vi "Duplicate.vi"(8 "error in":errorcluster, 10 "parameters":variant, 11 "DMM Channel in":refnum<class "DMM Channel.lvclass">) -> (0 "error out":errorcluster, 3 "DMM Channel out":refnum<class "DMM Channel.lvclass">)   [LabVIEW 2025, in "DMM.lvlib" / "DMM Channel.lvclass"]
doc: "Implements the specific behavior of a node when it is being duplicated\nCan be used to change the name of the new node for example adding Copy to it. \nCopyright 2017 National Instruments Corporation\n\nLicensed under the Apache License, Version 2.0 (the \"License\"); you may not use this file except in compliance with the License. You may obtain a copy of the License at http://www.apache.org/licenses/LICENSE-2.0\nUnless required by applicable law or agreed to in writing, software distributed under the License is distributed on an \"AS IS\" BASIS, WITHOUT WARRANTIES OR CONDITIONS OF ANY KIND, either express or implied. See the License for the specific language governing permissions and limitations under the License."
uses:
  DMM Channel.lvclass
  DMM Channel.lvclass/DMM Channel.ctl
  Users/Public/Documents/Sandia National Labs/TSS Plugin/Abstract Engine.lvlibp/Plugin/Abstract/Channel configuration/Read Channel Setting.vi
  Users/Public/Documents/Sandia National Labs/TSS Plugin/Abstract Engine.lvlibp/Plugin/Abstract/Channel configuration/Write Channel Setting.vi
  Users/Public/Documents/Sandia National Labs/TSS Plugin/Abstract Engine.lvlibp/Plugin/Abstract/Abstract Channel/Abstract Channel.lvclass
  Users/Public/Documents/Sandia National Labs/TSS Plugin/Abstract Engine.lvlibp/Plugin/Abstract/Channel configuration/Channel configuration.lvclass
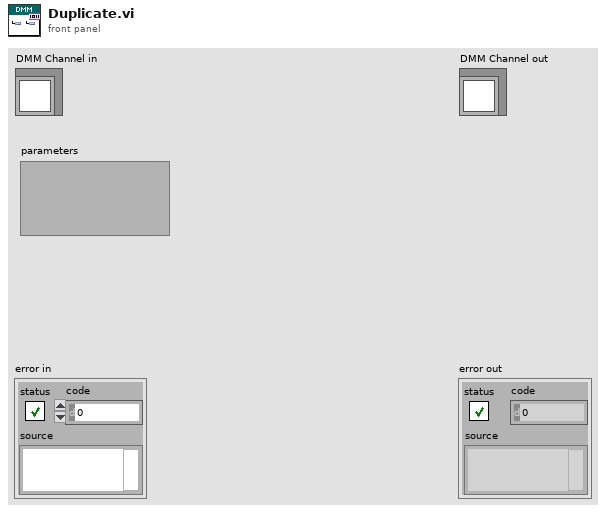
[diagram p1: front panel]
types:
  T1 = cluster{"Address":string, "SW Alias":string, "Description":string, "Enabled":bool, "Type":string}
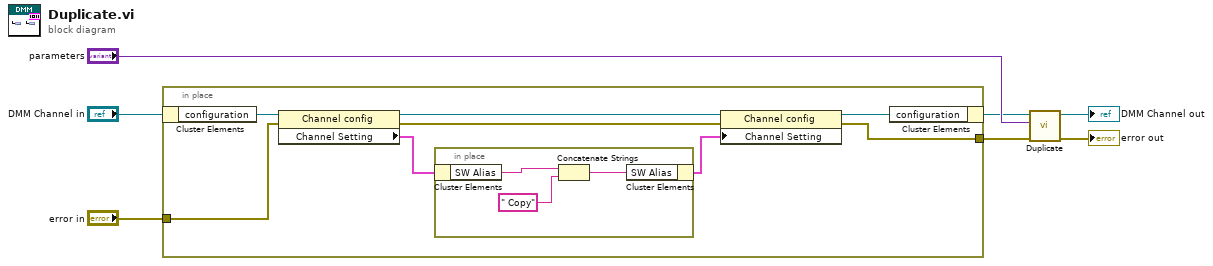
[diagram p0: block diagram]
diagram:
  n1 = in-place {
    in-place-border: "error in" -> [w10]
    in-place-border: [w8] -> w1
    n2 = in-place-cluster #1("DMM Channel in") -> ("configuration"=w15:refnum<class "Channel configuration.lvclass">)
    n3 = property class="Channel config"(reference=w15, error in=w10) -> (reference out=w14:refnum<class "Channel configuration.lvclass">, error out=w9:errorcluster, "Channel Setting"=w12:T1)
    n4 = in-place {
      n5 = in-place-cluster #2(w12) -> ("SW Alias"=w18:string)
      n6 = Concatenate Strings(w18, " Copy") -> (w17:string)
      n7 = in-place-cluster #2("SW Alias"=w17) -> (w11:T1)
    }
    n8 = property class="Channel config"(reference=w14, error in=w9, "Channel Setting"=w11) -> (reference out=w13:refnum<class "Channel configuration.lvclass">, error out=w8:errorcluster)
    n9 = in-place-cluster #1("configuration"=w13) -> (w3:refnum<class "DMM Channel.lvclass">)
  }
  n10 = call-parent "Duplicate.vi"("error in"=w1, "parameters"="parameters", "CEF_Serialize node in"=w3) -> ("error out"=→"error out":errorcluster, "CEF_Serialize node out"=→"DMM Channel out":refnum<class "DMM Channel.lvclass">)  [unwired: 7 in]
